vi "Apply Speed.vi"(8 "error in (no error)":errorcluster, 10 "Number of Points":i32, 11 "Tool Path in":refnum<class "Tool Path.lvclass">) -> (0 "error out":errorcluster, 2 "Speed Values":dbl[](array[numeric]), 3 "Tool Path out":refnum<class "Tool Path.lvclass">)   [LabVIEW 2019, in "Tool Path.lvclass"]
uses:
  Tool Path.lvclass
  subVIs/typedefs/Schedule Types/Schedule--Constant.ctl
  Settings/ObjectSettings/ObjectSettings.lvclass
  Settings/Path Settings/Path Settings.lvclass
  C:/Users/Albro/Documents/GitHub/AFM-Lithography/lvsrc/Classes/Settings/ObjectSettings/ObjectSettings.lvclass
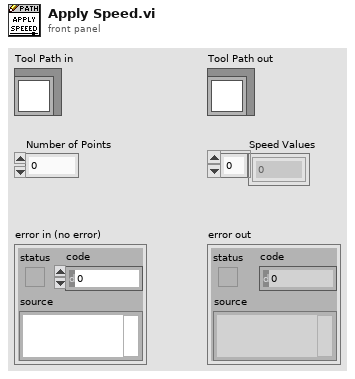
[diagram p1: front panel]
types:
  T1 = typedef "Schedule--Constant.ctl" = cluster{"Value":dbl}
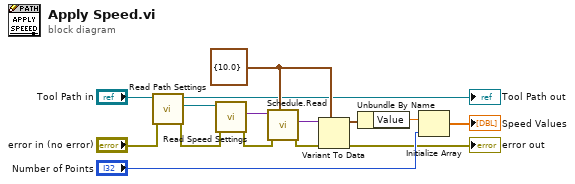
[diagram p0: block diagram]
diagram:
  w11 = T1 {"Value"=10.0} ("Constant")
  n1 = call-dynamic "Read Path Settings.vi"("error in (no error)"="error in (no error)", "Tool Path in"="Tool Path in") -> ("error out"=w3:errorcluster, "Path Settings.lvclass"=w4:refnum<class "Path Settings.lvclass">, "Tool Path out"=→"Tool Path out":refnum<class "Tool Path.lvclass">)  [unwired: 7 in]
  n2 = call "Read Speed Settings.vi"("error in (no error)"=w3, "ObjectSettings in"=w4) -> ("error out"=w2:errorcluster, "Settings"=w1:variant)  [unwired: 7 in, 1 out]
  n3 = call "Schedule.Read.vi"("Data to Read"=w11, "error in (no error)"=w2, "LUT In"=w1) -> ("error out"=w12:errorcluster, "Data Out"=w13:variant)  [unwired: 6 in, 1 out]
  n4 = Variant To Data(error in=w12, type=w11, Variant=w13) -> (data=w10:T1, error out=→"error out":errorcluster)
  n5 = Unbundle By Name(w10) -> ("Value"=w9:dbl)
  n6 = Initialize Array(w9, "Number of Points") -> (→"Speed Values":dbl[])
